vi "H.Signal.vi"() -> (4 "Slide servo home RS":bool, 6 "H.Signal":T1, 8 "LCD Pressing servo home RS":bool, 10 "Error Message":string, 15 "Bool_H Sig":bool)   [LabVIEW 2015]
uses:
  Galobal variable_TI.vi
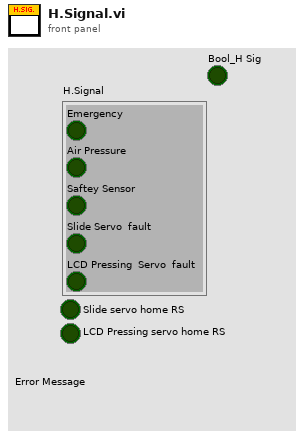
[diagram p1: front panel]
types:
  T1 = cluster{"Emergency":bool, "Air Pressure":bool, "Saftey Sensor":bool, "Slide Servo  fault":bool, "LCD Pressing  Servo  fault":bool}
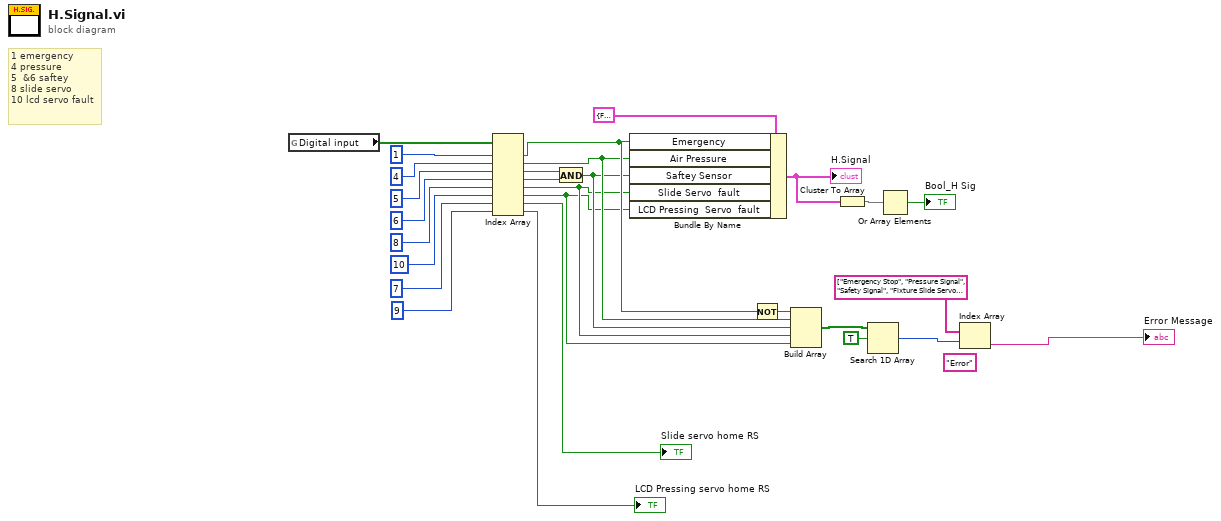
[diagram p0: block diagram]
diagram:
  (unwired) "Error" ("string")
  # "1 emergency\n4 pressure\n5  &6 saftey\n8 slide servo\n10 lcd servo fault"
  n1 = global read "Galobal variable_TI.vi" "Digital input"() -> (w28:bool[])
  n2 = Index Array(array=w28, index #1=1 ("index"), index #2=4 ("index"), index #3=5 ("index"), index #4=6 ("index"), index #5=8 ("index"), index #6=10 ("index"), index #7=7 ("index"), index #8=9 ("index")) -> (element #1=w14:bool, element #2=w12:bool, element #3=w21:bool, element #4=w20:bool, element #5=w10:bool, element #6=w9:bool, element #7=→"Slide servo home RS":bool, element #8=→"LCD Pressing servo home RS":bool)
  n3 = And(x=w21, y=w20) -> (x .and. y?=w11:bool)
  n4 = Bundle By Name(cluster=T1 {"Emergency"=FALSE, "Air Pressure"=FALSE, "Saftey Sensor"=FALSE, "Slide Servo  fault"=FALSE, "LCD Pressing  Servo  fault"=FALSE} ("Cluster"), "Emergency"=w14, "Air Pressure"=w12, "Saftey Sensor"=w11, "Slide Servo  fault"=w10, "LCD Pressing  Servo  fault"=w9) -> (w4:T1)
  "H.Signal" <- w4
  n5 = Not(x=w14) -> (.not. x?=w13:bool)
  n6 = Build Array(w13, w12, w11, w10, w9) -> (w15:bool[])
  n7 = Cluster To Array(cluster=w4) -> (array=w3:bool[])
  n8 = Search 1D Array(1D array=w15, element=TRUE) -> (index of element=w17:i32)  [unwired: 1 in]
  n9 = Or Array Elements(Boolean array=w3) -> (logical OR=→"Bool_H Sig":bool)
  n10 = Index Array(array=string[] ["Emergency Stop", "Pressure Signal", "Safety Signal", "Fixture Slide Servo Fault", "LCD Pressing Servo Fault"], index=w17) -> (element=→"Error Message":string)
